vi "settings.vi"(8 "error in (no error)":errorcluster, 11 "Template in":refnum<class "Template.lvclass">) -> (0 "error out":errorcluster, 3 "Template out":refnum<class "Template.lvclass">)   [LabVIEW 2020, in "Template.lvlib" / "Template.lvclass"]
uses:
  Template.lvclass
  Template.lvclass/Template.ctl
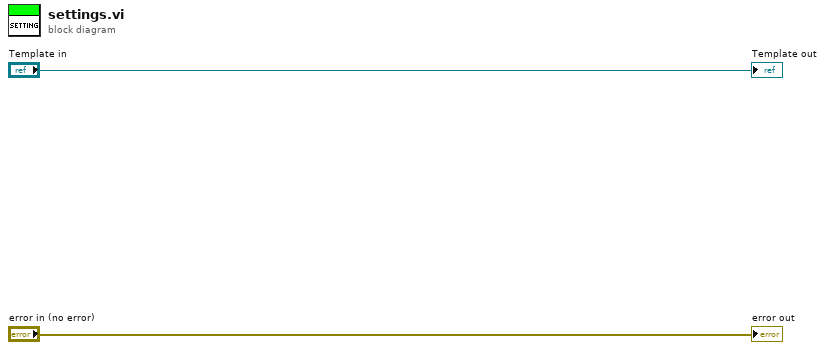
[diagram p0: block diagram]
diagram:
  "error out" <- "error in (no error)"
  "Template out" <- "Template in"
